vi "FPGA_Datalog_Main.vi"() -> ()   [LabVIEW 2018]
uses:
  <vilib>/rvi/Emulation/niFpgaGetClockAttributes.vi
  <vilib>/rvi/Emulation/niFpgaSctlEmulationGetInTimedLoop.vi
  <vilib>/rvi/Emulation/niFpgaEmulationReportErrorSimple.vi
  <vilib>/rvi/eio/common/nirviEmuTemplateMethod_errors.vi
  <vilib>/rvi/interface/RandomDataEmulation/niFpgaRandomDataHandleErrors.vi
  <vilib>/rvi/Emulation/niFpgaCriticalErrorInLSC.vi
  <vilib>/eio/EIONode/EIONode.xnode
  <vilib>/rvi/DataTransferAndStorage/Container/XNode/niFpgaContainer.xnode
  <vilib>/rvi/interface/RandomDataEmulation/nirviRandomDataFpgaReadWriteTemplate.vi
panel:
  in  "Actuation":u16
  in  "stop":bool
  in  "Acquisition Period (muS)":u32=2
  out "Measurement":u16
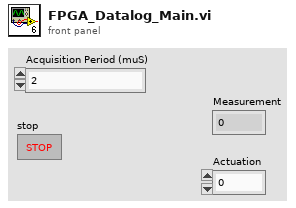
[diagram p1: front panel]
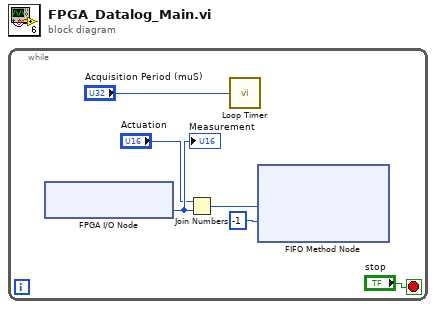
[diagram p0: block diagram]
diagram:
  n1 = while {
    stop <- "stop" stop-if-true
    n2 = xnode "FPGA I/O Node"() -> ("ConnectorB/AI0"=w4:u16)  [unwired: 1 in, 1 out]
    "Measurement" <- w4
    n3 = Join Numbers(hi="Actuation", lo=w4) -> ((hi.lo)=w3:u32)
    n4 = call "Loop Timer"("Count(uSec)"="Acquisition Period (muS)") -> ()  [unwired: 1 out]
    n5 = xnode ("FIFO Method Node")("Element"=w3, "Timeout"=-1) -> ()  [unwired: 1 in, 2 out]
  }
